vi "fpga.sandbox.vi"() -> ()   [LabVIEW 2020]
uses:
  orderbook/orderbook.command.data.ctl
  orderbook/orderbook.command.type.ctl
panel:
  out "x << y":u64 format="%.0x"
  out "output cluster":T1
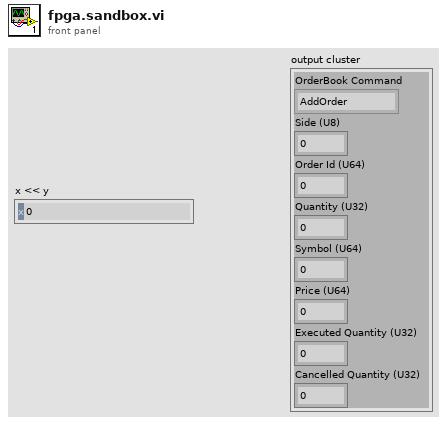
[diagram p1: front panel]
types:
  T1 = typedef "orderbook.command.data.ctl" = cluster{"OrderBook Command":T2, "Side (U8)":u8, "Order Id (U64)":u64, "Quantity (U32)":u32, "Symbol (U64)":u64, "Price (U64)":u64, "Executed Quantity (U32)":u32, "Cancelled Quantity (U32)":u32}
  T2 = typedef "orderbook.command.type.ctl" = enum16{"AddOrder", "OrderExecuted", "ReduceSize", "ModifyOrder", "DeleteOrder"}
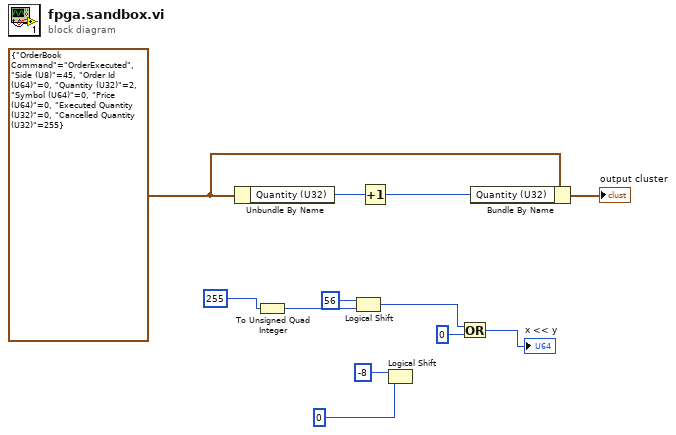
[diagram p0: block diagram]
diagram:
  w9 = T1 {"OrderBook Command"=enum."OrderExecuted", "Side (U8)"=45, "Order Id (U64)"=0, "Quantity (U32)"=2, "Symbol (U64)"=0, "Price (U64)"=0, "Executed Quantity (U32)"=0, "Cancelled Quantity (U32)"=255} ("Cluster")
  n1 = Unbundle By Name(w9) -> ("Quantity (U32)"=w11:u32)
  n2 = To Unsigned Quad Integer(1:u8 255 ("x")) -> (0:w6:u64)
  n3 = Logical Shift(y=i16 56, x=w6) -> (x << y=w3:u64)
  n4 = Increment(x=w11) -> (x+1=w10:u32)
  n5 = Logical Shift(y=i16 -8, x=u64 0) -> ()  [unwired: 1 out]
  n6 = Or(x=w3, y=u64 0) -> (x .or. y?=→"x << y":u64)
  n7 = Bundle By Name(cluster=w9, "Quantity (U32)"=w10) -> (→"output cluster":T1)
